vi "SetCorrelationId.vi"(8 "error in (no error)":errorcluster, 11 "header in":T1) -> (0 "error out":errorcluster, 2 "correlation Id":string, 3 "header out":T1)   [LabVIEW 2017]
uses:
  <vilib>/addons/InsightCM/MessageBus/Base/controls/MessageHeader.ctl
  <vilib>/addons/InsightCM/MessageBus/Base/controls/KeyValuePair.ctl
  <vilib>/addons/InsightCM/SRP/SRP.lvlib
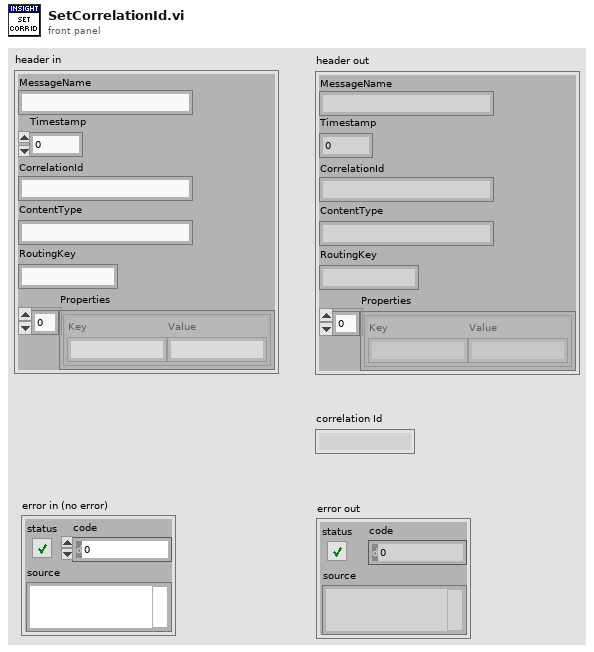
[diagram p1: front panel]
types:
  T1 = typedef "MessageHeader.ctl" = cluster{"MessageName":string, "Timestamp":i64, "CorrelationId":string, "ContentType":string, "RoutingKey":string, "Properties":T2[]}
  T2 = typedef "KeyValuePair.ctl" = cluster{"Key":string, "Value":string}
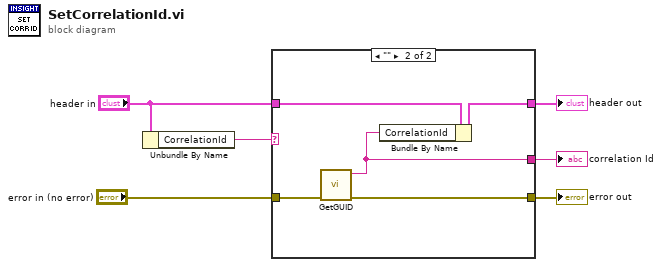
[diagram p0: block diagram]
diagram:
  n1 = Unbundle By Name("header in") -> ("CorrelationId"=w4:string)
  n2 = case shown="\"\"" w4 {
    tunnel: [w8 w13] -> w6
    tunnel: "header in" -> [w8 w12]
    tunnel: [_ w11] -> w3
    tunnel: "error in (no error)" -> [w7 w10]
    tunnel: [w7 w9] -> w1
    frame Default {
    }
    frame "" {
      n3 = call <vilib>:"GetGUID.vi"("error in (no error)"=w10) -> ("error out"=w9:errorcluster, "GUID"=w11:string)  [unwired: 9 in]
      n4 = Bundle By Name(cluster=w12, "CorrelationId"=w11) -> (w13:T1)
    }
  }
  "header out" <- w6
  "correlation Id" <- w3
  "error out" <- w1
